vi "SetFullSpeedTransfer.vi"(8 "error in (no error)":errorcluster, 10 "Tranfer speed":T1, 11 "ScopeBase In":refnum<class "ScopeBase.lvclass">) -> (0 "error out":errorcluster, 3 "ScopeBase Out":refnum<class "ScopeBase.lvclass">)   [LabVIEW 2025, in "ScopeBase.lvclass"]
uses:
  ScopeBase.lvclass
  controls/host_transfer_speed.ctl
  ScopeBase.lvclass/ScopeBase.ctl
  <vilib>/Utility/error.llb/Error Cluster From Error Code.vi
  <vilib>/rvi/errors/niLvFpgaAdjustHostInterfaceError.vi
  <vilib>/rvi/interface/nirviReadWriteControl/nirviReadWriteControl.xnode
  FpgaRef/FpgaRefBase/Common FPGA ref.ctl
  FpgaRef/FpgaRefBase/FpgaRefBase.lvclass
  NiFpgaLv.dll
  <vilib>/rvi/interface/Simulation/niFpgaSimulationCallBeginRW.vi
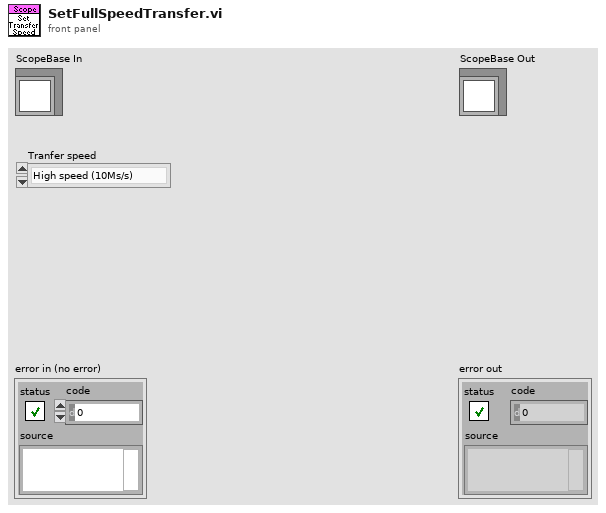
[diagram p1: front panel]
types:
  T1 = typedef "host_transfer_speed.ctl" = enum16{"High speed (10Ms/s)", "Low speed (1Ms/s)", "Ultra low speed (50kS/s)"}
  T2 = typedef "Common FPGA ref.ctl" = refnum<k20>
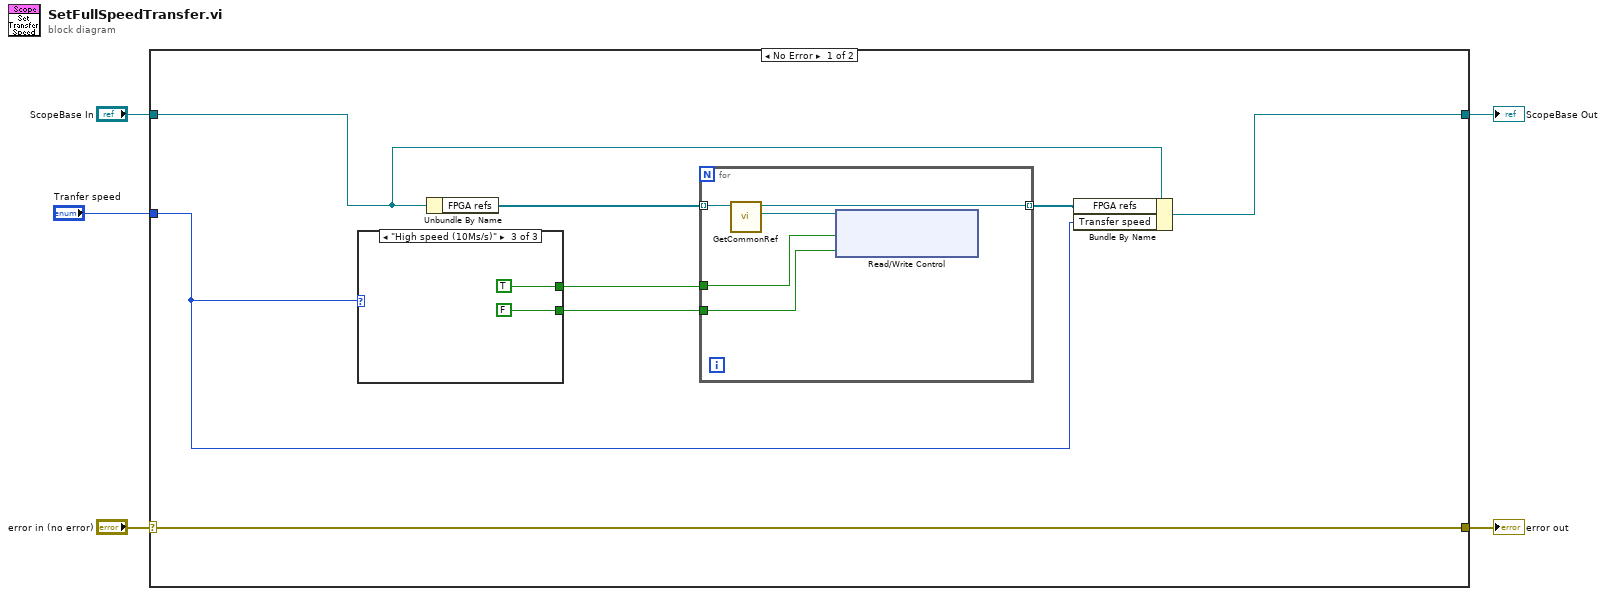
[diagram p0: block diagram]
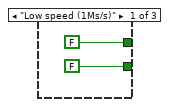
[diagram p2: hidden frame]
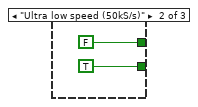
[diagram p3: hidden frame]
diagram:
  n1 = case shown="No Error" "error in (no error)" {
    selector: "error in (no error)" -> [w13 w26]
    tunnel: [w13 w26] -> w3
    tunnel: [w10 w25] -> w4
    tunnel: "ScopeBase In" -> [w9 w25]
    tunnel: "Tranfer speed" -> [w6 _]
    frame No Error {
      n2 = case shown="\"High speed (10Ms/s)\"" w6 {
        tunnel: [FALSE FALSE TRUE] -> w8
        tunnel: [FALSE TRUE FALSE] -> w7
        frame "Low speed (1Ms/s)" {
        }
        frame "Ultra low speed (50kS/s)" {
        }
        frame "High speed (10Ms/s)" {
        }
      }
      n3 = Unbundle By Name(w9) -> ("FPGA refs"=w12:refnum<class "FpgaRefBase.lvclass">[])
      n4 = for {
        tunnel: w8 -> [w24]
        tunnel: w12 -> [w23] mode=indexing
        tunnel: [w21] -> w11 mode=indexing
        tunnel: w7 -> [w20]
        n5 = call-dynamic "GetCommonRef.vi"("FpgaRefBase in"=w23) -> ("Common ref"=w22:T2, "FpgaRefBase out"=w21:refnum<class "FpgaRefBase.lvclass">)  [unwired: 8 in, 1 out]
        n6 = xnode "Read/Write Control"("FPGA VI Reference In"=w22, "Full speed transfer"=w24, "Ultra low speed transfer"=w20) -> ()  [unwired: 1 in, 2 out]
      }
      n7 = Bundle By Name(cluster=w9, "FPGA refs"=w11, "Transfer speed"=w6) -> (w10:refnum<class "ScopeBase.lvclass">)
    }
    frame Error {
    }
  }
  "error out" <- w3
  "ScopeBase Out" <- w4
